vi "Test SUBSCRIBE packet.vi"(8 "error in (no error)":errorcluster) -> (0 "error out":errorcluster)   [LabVIEW 2013]
uses:
  source/Control Packets/SUBSCRIBE/Topic Subscription -- cluster.ctl
  source/Control Packets/ControlPacket/QualityOfService -- enum.ctl
  source/Control Packets/SUBSCRIBE/SUBSCRIBE.lvclass
  source/Control Packets/ControlPacket/ControlPacket.lvclass/ControlPacket.ctl
  source/Control Packets/ControlPacket/ControlPacket.lvclass
  <vilib>/addons/_JKI Toolkits/Caraya/classes/Test/Test.lvclass
  <vilib>/addons/_JKI Toolkits/Caraya/classes/Assert/Assert.lvclass
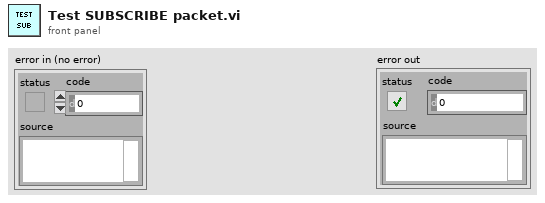
[diagram p1: front panel]
types:
  T1 = typedef "MQTT_Control_Packets.lvlib/SUBSCRIBE.lvclass/Topic Subscription -- cluster.ctl" = cluster{"Topic Filter":string, "QoS":T2}
  T2 = typedef "MQTT_Control_Packets.lvlib/ControlPacket.lvclass/QualityOfService -- enum.ctl" = enum16{"0 (At Most Once)", "1 (At Least Once)", "2 (Exactly Once)"}
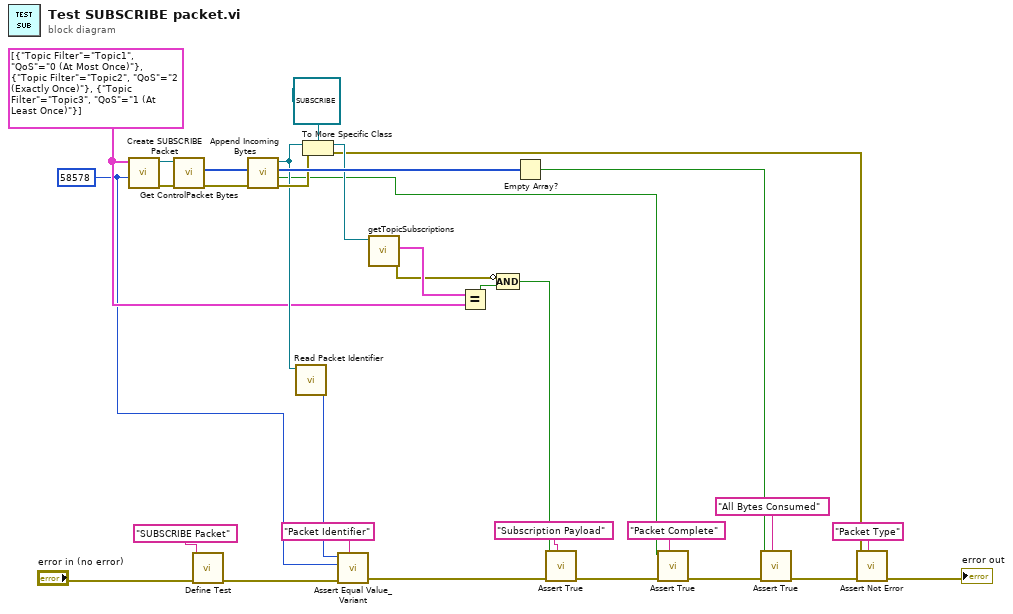
[diagram p0: block diagram]
diagram:
  w25 = T1[] [{"Topic Filter"="Topic1", "QoS"=enum."0 (At Most Once)"}, {"Topic Filter"="Topic2", "QoS"=enum."2 (Exactly Once)"}, {"Topic Filter"="Topic3", "QoS"=enum."1 (At Least Once)"}] ("Topic Subscriptions")
  w9 = u16 58578 ("Packet ID")
  n1 = call "Create SUBSCRIBE Packet.vi"("Packet ID (empty: Generate new)"=w9, "Topic Subscriptions"=w25) -> ("error out"=w26:errorcluster, "SUBSCRIBE out"=w27:refnum<class "SUBSCRIBE.lvclass">)  [unwired: 8 in]
  n2 = call "Get ControlPacket Bytes.vi"("error in (no error)"=w26, "ControlPacket"=w27) -> ("error out"=w30:errorcluster, "Bytes Stream"=w32:u8[])  [unwired: 6 in, 2 out]
  n3 = call <vilib>:"Define Test.vi"("error in (no error)"="error in (no error)", "Label (VI Title)"="SUBSCRIBE Packet") -> ("error out"=w14:errorcluster)  [unwired: 9 in]
  n4 = call "Append Incoming Bytes.vi"("error in (no error)"=w30, "Incoming Packets"=w32) -> ("error out"=w29:errorcluster, "Complete Packet"=w5:bool, "Remaining Packets"=w31:u8[], "ControlPacket"=w28:refnum<class "ControlPacket.lvclass">)  [unwired: 6 in]
  n5 = call "Read Packet Identifier.vi"("ControlPacket in"=w28) -> ("Packet Identifier"=w8:u16)  [unwired: 9 in, 1 out]
  n6 = To More Specific Class(target class=refnum<class "SUBSCRIBE.lvclass"> refnum ("MQTT_Control_Packets.lvlib:SUBSCRIBE.lvclass"), reference=w28, error in=w29) -> (specific class reference=w24:refnum<class "SUBSCRIBE.lvclass">, error out=w7:errorcluster)
  n7 = call <vilib>:"Assert Equal Value_Variant.vi"("Label"="Packet Identifier" ("Label (VI Title)"), "error in (no error)"=w14, "Y"=w9, "X"=w8) -> ("error out"=w3:errorcluster)  [unwired: 7 in]
  n8 = call "getTopicSubscriptions.vi"("SUBSCRIBE in"=w24) -> ("error out"=w22:errorcluster, "Topic Subscriptions"=w23:T1[])  [unwired: 8 in, 1 out]
  n9 = Equal?(x=w23, y=w25) -> (x = y?=w21:bool)
  n10 = Compound Arithmetic op=AND(invert w22, w21) -> (w1:bool)
  n11 = Empty Array?(array=w31) -> (empty?=w6:bool)
  n12 = call <vilib>:"Assert True.vi"("Label"="Subscription Payload" ("Label (VI Title)"), "error in (no error)"=w3, "True?"=w1) -> ("error out"=w2:errorcluster)  [unwired: 8 in]
  n13 = call <vilib>:"Assert True.vi"("Label"="Packet Complete" ("Label (VI Title)"), "error in (no error)"=w2, "True?"=w5) -> ("error out"=w15:errorcluster)  [unwired: 8 in]
  n14 = call <vilib>:"Assert True.vi"("Label"="All Bytes Consumed" ("Label (VI Title)"), "error in (no error)"=w15, "True?"=w6) -> ("error out"=w12:errorcluster)  [unwired: 8 in]
  n15 = call <vilib>:"Assert Not Error.vi"("Label"="Packet Type" ("Label (VI Title)"), "error in (no error)"=w12, "Not Error?"=w7) -> ("error out"=→"error out":errorcluster)  [unwired: 8 in]
